vi "testUpload.vi"() -> ()   [LabVIEW 2025]
uses:
  ocr/ocr.lvclass
  tcv/def/lvImgptrtoupload.ctl
  tcv/tcv.lvclass
panel:
  in  "stop":bool
  in  "Y Coordinate":i32
  in  "X Coordinate":i32
  out "Image":T1(plugin-control)
  in  "device":enum16{"CPU", "GPU0"}(ring)=enum."GPU0"
  out "error out":errorcluster
  out "SetDevice":string
  out "loadedImgSucc":i32
  in  "PathImage":path=path "D:/Test/dllTest/images/old"
  # "D:\\Test\\dllTest\\images\\old"
  # "D:\\Test\\dllTest\\images_2"
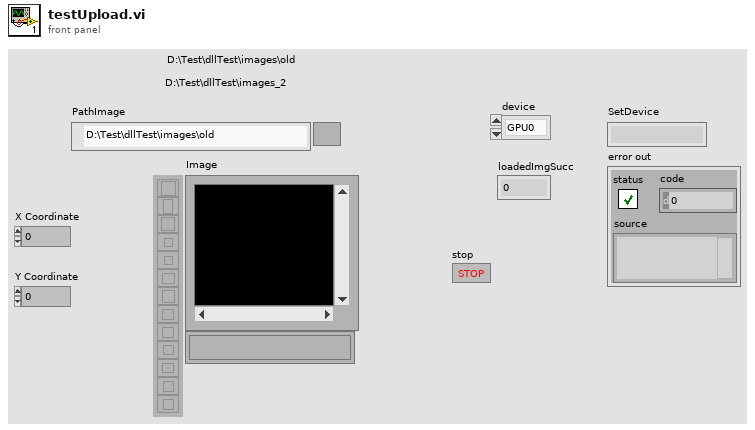
[diagram p1: front panel]
types:
  T1 = typedef "IMAQ Image.ctl" = refnum<image>
  T2 = typedef "tcv.lvlib/tcv.lvclass/lvImgptrtoupload.ctl" = cluster{"lvImgPtr":u64, "linewidth":i32, "height":i32, "width":i32}
  T3 = enum32{"Map Pixel Pointer", "Unmap Pixel Pointer", "Get Pixels Infos"}
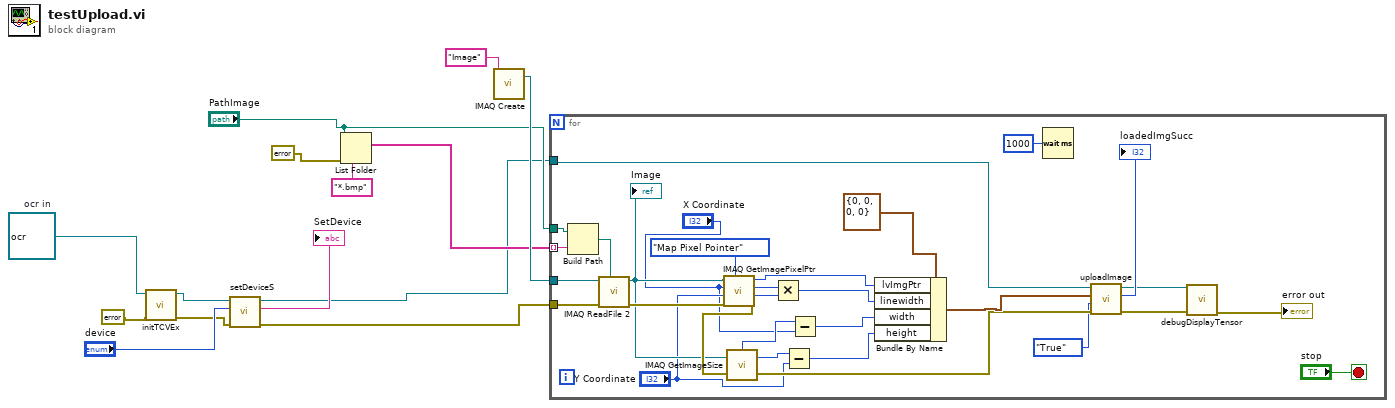
[diagram p0: block diagram]
diagram:
  w5 = refnum<class "ocr.lvclass"> refnum  # ocr in
  n1 = call-dynamic "initTCVEx.vi"("error in (no error)"=errorcluster {"status"=FALSE, "code"=0, "source"=""}, "tcv in"=w5) -> ("error out"=w2:errorcluster, "tcv out"=w4:refnum<class "ocr.lvclass">)  [unwired: 8 in]
  n2 = call-dynamic "setDeviceS.vi"("error in (no error)"=w2, "devices"="device", "tcv in"=w4) -> ("error out"=w1:errorcluster, "SetDevice"=→"SetDevice":string, "tcv out"=w6:refnum<class "ocr.lvclass">)  [unwired: 6 in]
  n3 = List Folder(path="PathImage", pattern="*.bmp", error in=errorcluster {"status"=FALSE, "code"=0, "source"=""}) -> (filenames=w8:string[])  [unwired: 1 in, 3 out]
  n4 = call "IMAQ Create"("Image Name"="Image") -> ("New Image"=w14:T1)  [unwired: 4 in, 1 out]
  n5 = for {
    tunnel: "PathImage" -> [w44]
    tunnel: w14 -> [w42]
    tunnel: w8 -> [w35] mode=indexing
    tunnel: w6 -> [w32]
    tunnel: w1 -> [w15]
    stop <- "stop" stop-if-true
    n6 = Build Path(base path=w44, name or relative path=w35) -> (appended path=w43:path)
    n7 = call "IMAQ ReadFile 2"("File Path"=w43, "error in (no error)"=w15, "Image"=w42) -> ("error out"=w41:errorcluster, "Image Out"=w27:T1)  [unwired: 4 in, 3 out]
    "Image" <- w27
    n8 = call "IMAQ GetImagePixelPtr"("Function"=T3."Map Pixel Pointer", "error in (no error)"=w41, "Y Coordinate"="Y Coordinate", "X Coordinate"="X Coordinate", "Image"=w27) -> ("error out"=w39:errorcluster, "Pixel Size (Bytes)"=w37:i32, "LineWidth(Pixels)"=w38:i32, "Pixel Pointer out"=w34:u64)  [unwired: 1 in, 2 out]
    n9 = call "IMAQ GetImageSize"("Image"=w27, "error in (no error)"=w39) -> ("Y Resolution"=w22:i32, "X Resolution"=w19:i32, "error out"=w30:errorcluster)  [unwired: 2 in]
    n10 = Multiply(x=w38, y=w37) -> (x*y=w33:i32)
    n11 = Subtract(x=w22, y="Y Coordinate") -> (x-y=w20:i32)
    n12 = Subtract(x=w19, y="X Coordinate") -> (x-y=w17:i32)
    n13 = Bundle By Name(cluster=T2 {"lvImgPtr"=0, "linewidth"=0, "height"=0, "width"=0} ("lvImgptrtoupload"), "lvImgPtr"=w34, "linewidth"=w33, "width"=w17, "height"=w20) -> (w31:T2)
    n14 = Wait (ms)(milliseconds to wait=u32 1000) -> ()  [unwired: 1 out]
    n15 = call-dynamic "uploadImage.vi"("error in (no error)"=w30, "Normalize"=enum16{"False", "True"}."True", "lvImgptrtoupload"=w31, "tcv in"=w32) -> ("error out"=w26:errorcluster, "uploadImgSucc"=→"loadedImgSucc":i32, "tcv out"=w24:refnum<class "ocr.lvclass">)  [unwired: 2 in, 1 out]
    n16 = call-dynamic "debugDisplayTensor.vi"("error in (no error)"=w26, "tcv in"=w24) -> ("error out"=→"error out":errorcluster)  [unwired: 6 in, 3 out]
  }
